vi "Create.vi"(8 "error in (no error)":errorcluster, 11 "ICPCON ET-7017 in":refnum<class "ICPCON ET-7017-10.lvclass">) -> (0 "error out":errorcluster, 3 "ICPCON ET-7017 out":refnum<class "ICPCON ET-7017-10.lvclass">)   [LabVIEW 2021, in "ICPCON ET-7017-10.lvclass"]
uses:
  ICPCON ET-7017-10.lvclass
  D:/my_projects/projects/Algorithms/Labview/21/Modbus_v121c/Network Protocol/MB/Modbus Master CR.lvclass
  Data Model/ICPCON ET7000 Data Model/ET-7017-10/ET-7017-10 Data Model.lvclass
  D:/my_projects/projects/Algorithms/Labview/21/Modbus_v121c/Data Model/Device Data Model.lvclass
  MB/Modbus Master CR.lvclass/Modbus Master CR.ctl
  TCP/TCP.lvclass
  MB/Modbus Master CR.lvclass
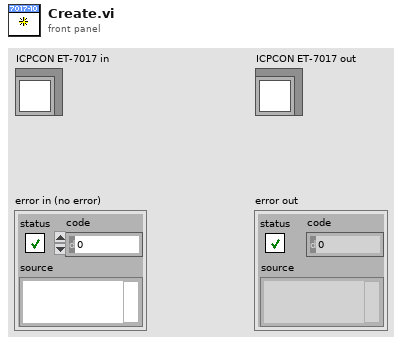
[diagram p1: front panel]
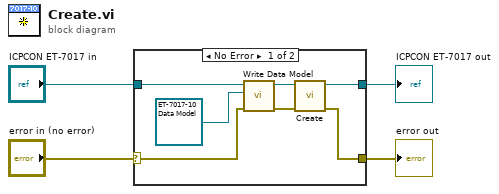
[diagram p0: block diagram]
diagram:
  n1 = case shown="No Error" "error in (no error)" {
    selector: "error in (no error)" -> [w5 w12]
    tunnel: [w9 w12] -> w1
    tunnel: [w10 w13] -> w2
    tunnel: "ICPCON ET-7017 in" -> [w11 w13]
    frame No Error {
      n2 = call "Write Data Model.vi"("error in (no error)"=w5, "Data Model"=refnum<class "ET-7017-10 Data Model.lvclass"> refnum ("Modbus API:Device Data Model"), "MB_TCP in"=w11) -> ("error out"=w8:errorcluster, "MB_TCP out"=w7:refnum<class "ICPCON ET-7017-10.lvclass">)  [unwired: 7 in]
      n3 = call-parent "Create.vi"("error in (no error)"=w8, "TCP in"=w7) -> ("error out"=w9:errorcluster, "TCP out"=w10:refnum<class "ICPCON ET-7017-10.lvclass">)  [unwired: 8 in]
    }
    frame Error {
    }
  }
  "error out" <- w1
  "ICPCON ET-7017 out" <- w2
